vi "OpenVS(Silent).vi"(11 "Silent VeriStand?":bool) -> ()   [LabVIEW 2013, in "MiscHelperVIs.lvlib"]
uses:
  MiscHelperVIs.lvlib
  <vilib>/Utility/sysdir.llb/System Directory Type.ctl
panel:
  # "This VI calls VS silently if passed a True"
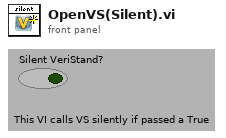
[diagram p1: front panel]
types:
  T1 = typedef "System Directory Type.ctl" = i32
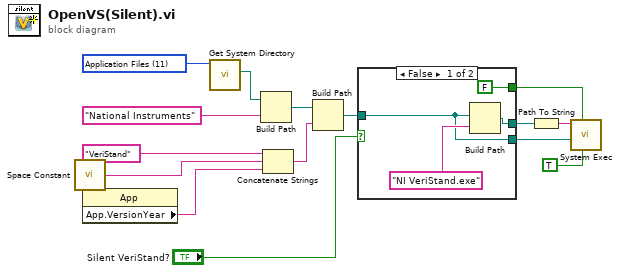
[diagram p0: block diagram]
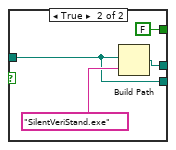
[diagram p2: hidden frame]
diagram:
  w14 = T1 11 items=["User Home"=0, "User Desktop"=1, "User Documents"=2, "User Application Data"=3, "User Preferences"=4, "User Temporary"=5, "Public Documents"=6, "Public Application Data"=7, "Public Preferences"=8, "Public Cache"=13, "System Core Libraries"=9, "System Installed Libraries"=10, "Application Files"=11, "Boot Volume Root"=12] ("system directory type")
  n1 = call <vilib>:"Space Constant.vi"() -> ("String"=w5:string)
  n2 = property class="App"() -> ("App.VersionYear"=w6:string)  [unwired: 2 in, 2 out]
  n3 = call <vilib>:"Get System Directory.vi"("system directory type"=w14) -> ("system directory"=w13:path)  [unwired: 10 in]
  n4 = Build Path(base path=w13, name or relative path="National Instruments") -> (appended path=w11:path)
  n5 = Concatenate Strings("VeriStand" ("name or relative path"), w5, w6) -> (w4:string)
  n6 = Build Path(base path=w11, name or relative path=w4) -> (appended path=w8:path)
  n7 = case shown="False" "Silent VeriStand?" {
    tunnel: [w18 w22] -> w10
    tunnel: w8 -> [w17 w21]
    tunnel: [w17 w21] -> w2
    tunnel: [FALSE ("wait until completion? (T)") FALSE ("wait until completion? (T)")] -> w1
    frame False {
      n8 = Build Path(base path=w17, name or relative path="NI VeriStand.exe") -> (appended path=w18:path)
    }
    frame True {
      n9 = Build Path(base path=w21, name or relative path="SilentVeriStand.exe") -> (appended path=w22:path)
    }
  }
  n10 = Path To String(path=w10) -> (string=w9:string)
  n11 = call <vilib>:"System Exec.vi"("run minimized? (F)"=TRUE, "wait until completion? (T)"=w1, "working directory"=w2, "command line"=w9) -> ()  [unwired: 4 in, 4 out]
